vi "ReadPattern.vi"(0 "file path (dialog if empty)":path=path "C:/Users/Aerotech/Documents/BNL_ThermomechanicalStave/SchillaciGlue/GluePatterns/pattern.txt") -> (1 "Relative Line\nSeparations [mm]":dbl[][](array[numeric]), 2 "Line Lengths [mm]":dbl[](array[numeric]), 3 "Motion Time [s]":dbl[](array[numeric]), 4 "N Lines":i32)   [LabVIEW 2016]
uses:
  <vilib>/Utility/file.llb/Read Delimited Spreadsheet (DBL).vi
panel:
  out "all rows":dbl[][](array[numeric])
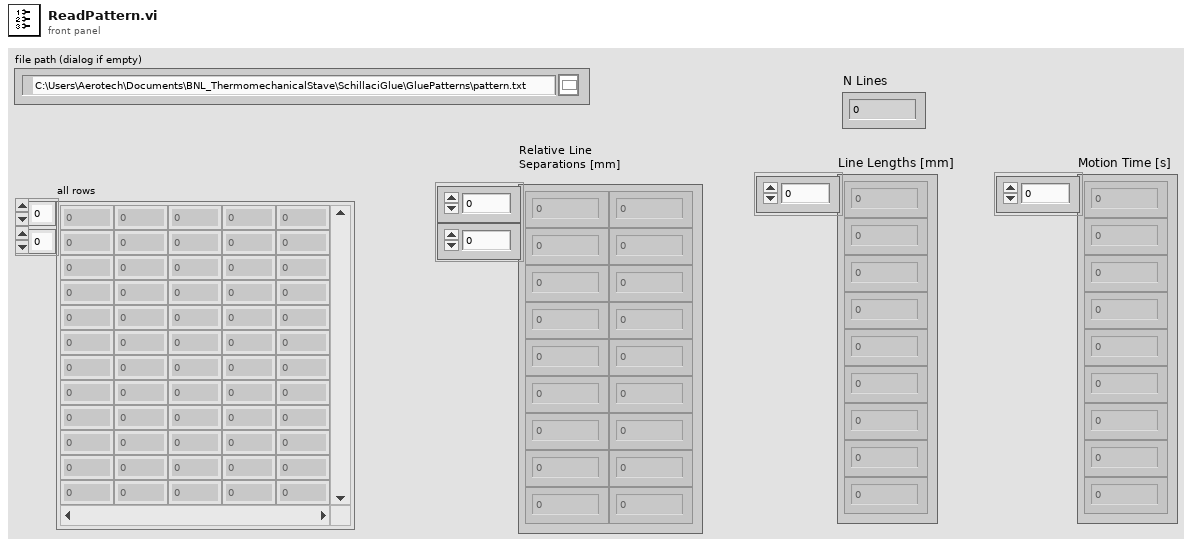
[diagram p1: front panel]
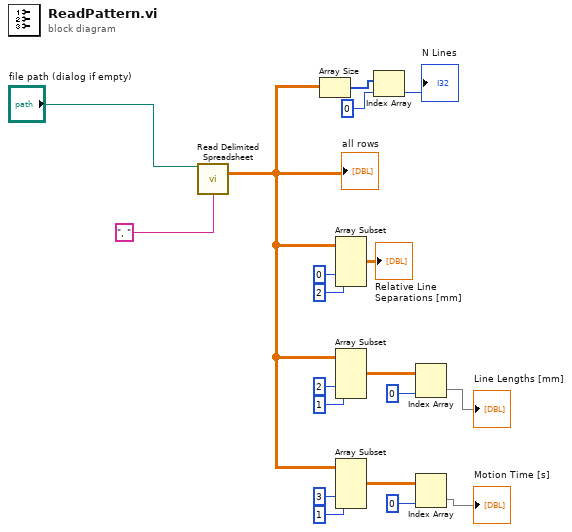
[diagram p0: block diagram]
diagram:
  n1 = call-poly <vilib>:"Read Delimited Spreadsheet.vi"("file path (dialog if empty)"="file path (dialog if empty)", "delimiter (\\t)"=", " ("delimiter (\\t)")) -> ("all rows"=w2:dbl[][])  [unwired: 8 in, 5 out]
  "all rows" <- w2
  n2 = Array Size(array=w2) -> (size(s)=w12:i32[])
  n3 = Array Subset(array=w2, index (col)=0 ("index"), length (col)=2 ("length")) -> (→"Relative Line\nSeparations [mm]":dbl[][])  [unwired: 2 in]
  n4 = Array Subset(array=w2, index (col)=2 ("index"), length (col)=1 ("length")) -> (w9:dbl[][])  [unwired: 2 in]
  n5 = Array Subset(array=w2, index (col)=3 ("index"), length (col)=1 ("length")) -> (w4:dbl[][])  [unwired: 2 in]
  n6 = Index Array(array=w12, index=0) -> (element=→"N Lines":i32)
  n7 = Index Array(array=w9, index (col)=0 ("disabled index (col)")) -> (element=→"Line Lengths [mm]":dbl[])  [unwired: 1 in]
  n8 = Index Array(array=w4, index (col)=0 ("disabled index (col)")) -> (element=→"Motion Time [s]":dbl[])  [unwired: 1 in]
